vi "Cooling-PID.vi"() -> (3 "appended array":digitalwaveform[](array[waveform]))   [LabVIEW 2020]
uses:
  <vilib>/Waveform/DWDTOps.llb/DWDT Analog to Digital.vi
  <vilib>/measure/NI_MABase.lvlib
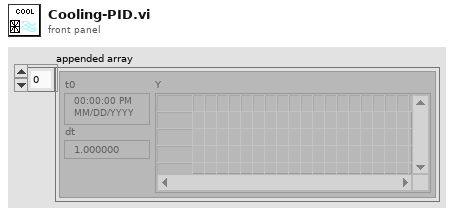
[diagram p1: front panel]
types:
  T1 = enum16{"Sine Wave", "Triangle Wave", "Square Wave", "Sawtooth Wave"}
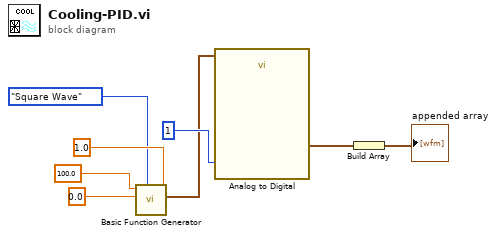
[diagram p0: block diagram]
diagram:
  n1 = call <vilib>:"Basic Function Generator.vi"("offset"=1.0, "signal type"=T1."Square Wave", "amplitude"=0.0, "frequency"=100.0) -> ("signal out"=w5:waveform(dbl))  [unwired: 5 in, 2 out]
  n2 = call-poly <vilib>:"Analog to Digital.vi"("resolution (16 bit)"=1, "analog waveform"=w5) -> ("digital waveform"=w6:digitalwaveform)  [unwired: 6 in, 3 out]
  n3 = Build Array(w6) -> (→"appended array":digitalwaveform[])
